vi "Reserve Hardware for DAQmx Task.vi"(7 "timeout, ms (10000)":u32=10000, 8 "error in (no error)":errorcluster, 11 "task/channels in":refnum<k21>) -> (0 "error out":errorcluster, 3 "task out":refnum<k21>)   [LabVIEW 2015, in "PL Utility.lvlib"]
doc: "Attempts to reserve the hardware resources needed for the DAQmx task with a specified <b>timeout</b>."
uses:
  PL Utility.lvlib
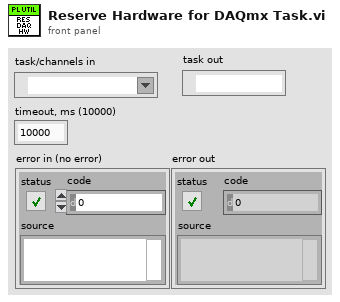
[diagram p1: front panel]
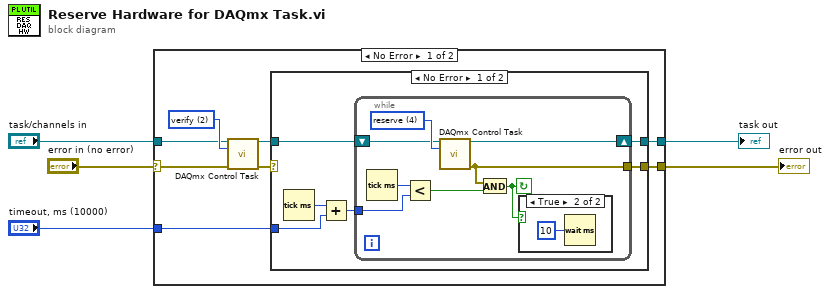
[diagram p0: block diagram]
diagram:
  n1 = case shown="No Error" "error in (no error)" {
    selector: "error in (no error)" -> [w13 w31]
    tunnel: [w7 w31] -> w4
    tunnel: "task/channels in" -> [w11 w32]
    tunnel: [w8 w32] -> w2
    tunnel: "timeout, ms (10000)" -> [w6 _]
    frame No Error {
      w12 = 2 items=["verify"=2, "reserve"=4, "commit"=3, "unreserve"=5, "abort"=6] ("action")
      n2 = call <vilib>:"DAQmx Control Task.vi"("task/channels in"=w11, "action"=w12, "error in"=w13) -> ("task out"=w9:refnum<k21>, "error out"=w10:errorcluster)  [unwired: 11 in]
      n3 = case shown="No Error" w10 {
        selector: w10 -> [_ w29]
        tunnel: w9 -> [w19 w30]
        tunnel: [w14 w30] -> w8
        tunnel: [w15 w29] -> w7
        tunnel: w6 -> [w16 _]
        frame No Error {
          n4 = Tick Count (ms)() -> (millisecond timer value=w17:u32)
          n5 = Add(x=w17, y=w16) -> (x+y=w18:u32)
          n6 = while {
            tunnel: w18 -> [w24]
            shift-right: [w22] -> w14
            shift-left: w19 -> [w26]
            tunnel: [w21] -> w15
            stop <- w20 continue-if-true
            w27 = 4 items=["verify"=2, "reserve"=4, "commit"=3, "unreserve"=5, "abort"=6] ("action")
            n7 = Tick Count (ms)() -> (millisecond timer value=w25:u32)
            n8 = Less?(x=w25, y=w24) -> (x < y?=w23:bool)
            n9 = call <vilib>:"DAQmx Control Task.vi"("task/channels in"=w26, "action"=w27) -> ("task out"=w22:refnum<k21>, "error out"=w21:errorcluster)  [unwired: 12 in]
            n10 = And(x=w21, y=w23) -> (x .and. y?=w20:bool)
            n11 = case shown="True" w20 {
              frame False {
              }
              frame True {
                n12 = Wait (ms)(milliseconds to wait=u32 10) -> ()  [unwired: 1 out]
              }
            }
          }
        }
        frame Error {
        }
      }
    }
    frame Error {
    }
  }
  "error out" <- w4
  "task out" <- w2
